vi "MeasureIVandCap.vi"(0 ".NET Refnum in":refnum<k24>, 1 ".NET Refnum":refnum<k24>, 2 "Junction Name":string, 5 "CurrentPositionIndex":i32, 7 "appended path":path, 9 "Numeric":dbl, 12 "new file path (Not A Path if cancelled)":path, 13 "UiDefinition":T1, 14 "Function":string) -> (15 "error out":errorcluster)   [LabVIEW 2020]
uses:
  C:/Users/User/Desktop/Automation/CurrentVersion/LabviewDXFViewer/bin/Release/LabviewDXFViewer.exe
  LabviewDXFViewer/bin/Release/LabviewDXFViewer.exe
  UIReferences.ctl
  <vilib>/Utility/file.llb/Write Delimited Spreadsheet (string).vi
  <vilib>/Utility/file.llb/Write Delimited Spreadsheet (DBL).vi
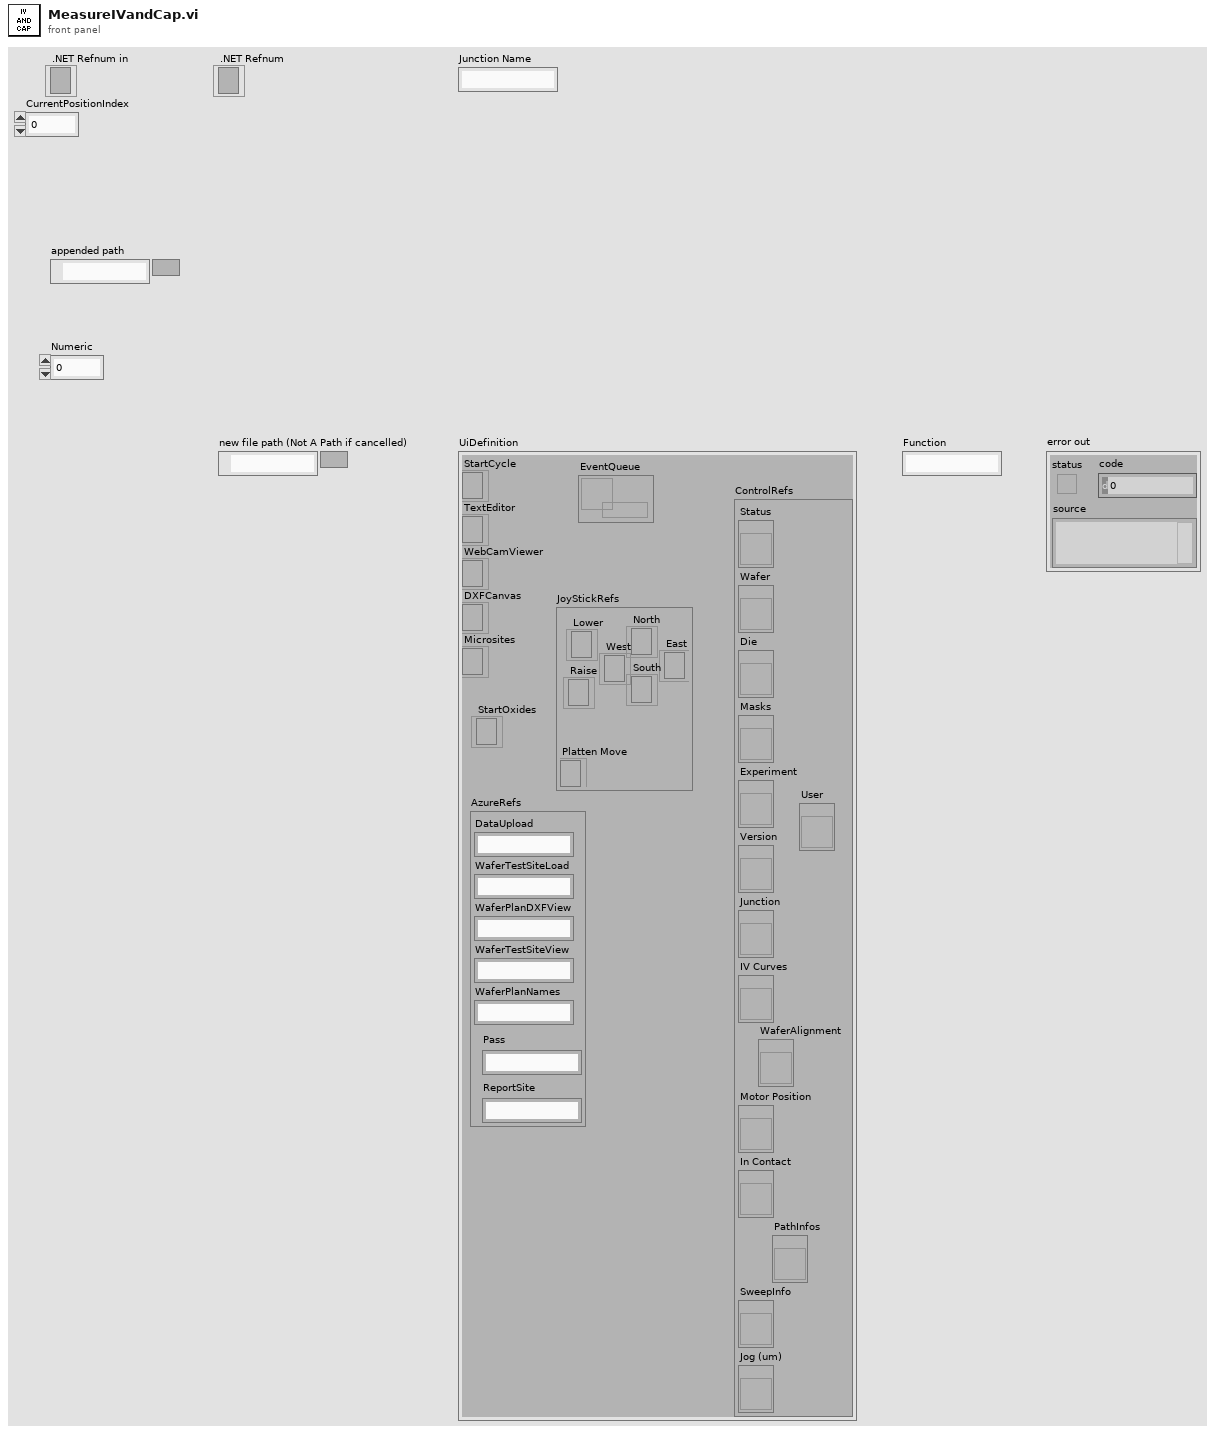
[diagram p1: front panel]
types:
  T1 = typedef "UIReferences.ctl" = cluster{"StartCycle":refnum<k24>, "TextEditor":refnum<k24>, "WebCamViewer":refnum<k24>, "DXFCanvas":refnum<k24>, "Microsites":refnum<k24>, "JoyStickRefs":cluster{"North":refnum<k24>, "Lower":refnum<k24>, "Raise":refnum<k24>, "Platten Move":refnum<k24>, "West":refnum<k24>, "East":refnum<k24>, "South":refnum<k24>}, "AzureRefs":cluster{"DataUpload":string, "WaferTestSiteLoad":string, "WaferPlanDXFView":string, "WaferTestSiteView":string, "WaferPlanNames":string, "Pass":string, "ReportSite":string}, "ControlRefs":cluster{"Status":refnum<vi>, "Wafer":refnum<vi>, "Die":refnum<vi>, "Masks":refnum<vi>, "Experiment":refnum<vi>, "Version":refnum<vi>, "Junction":refnum<vi>, "IV Curves":refnum<vi>, "Motor Position":refnum<vi>, "In Contact":refnum<vi>, "SweepInfo":refnum<vi>, "Jog (um)":refnum<vi>, "PathInfos":refnum<vi>, "User":refnum<vi>, "WaferAlignment":refnum<vi>}, "EventQueue":refnum<queue>, "StartOxides":refnum<k24>}
  T2 = typedef "CapacitanceInfos.ctl" = cluster{"Conductance":dbl, "CapacitanceIV":dbl, "Intercept":dbl, "CapacitanceSW":dbl, "Sum":dbl, "CapacitanceInfos":T3[], "CapacitancePhase":dbl, "dC/dV":dbl, "Function":string, "OtherInfo":dbl[][]}
  T3 = typedef "CapacitanceRecord.ctl" = cluster{"Freq":dbl, "Vpp":dbl, "PhaseS":dbl, "Irms":dbl, "PhaseC":dbl, "Theta":dbl, "VDrive":dbl, "Capacitance":dbl, "Other":dbl}
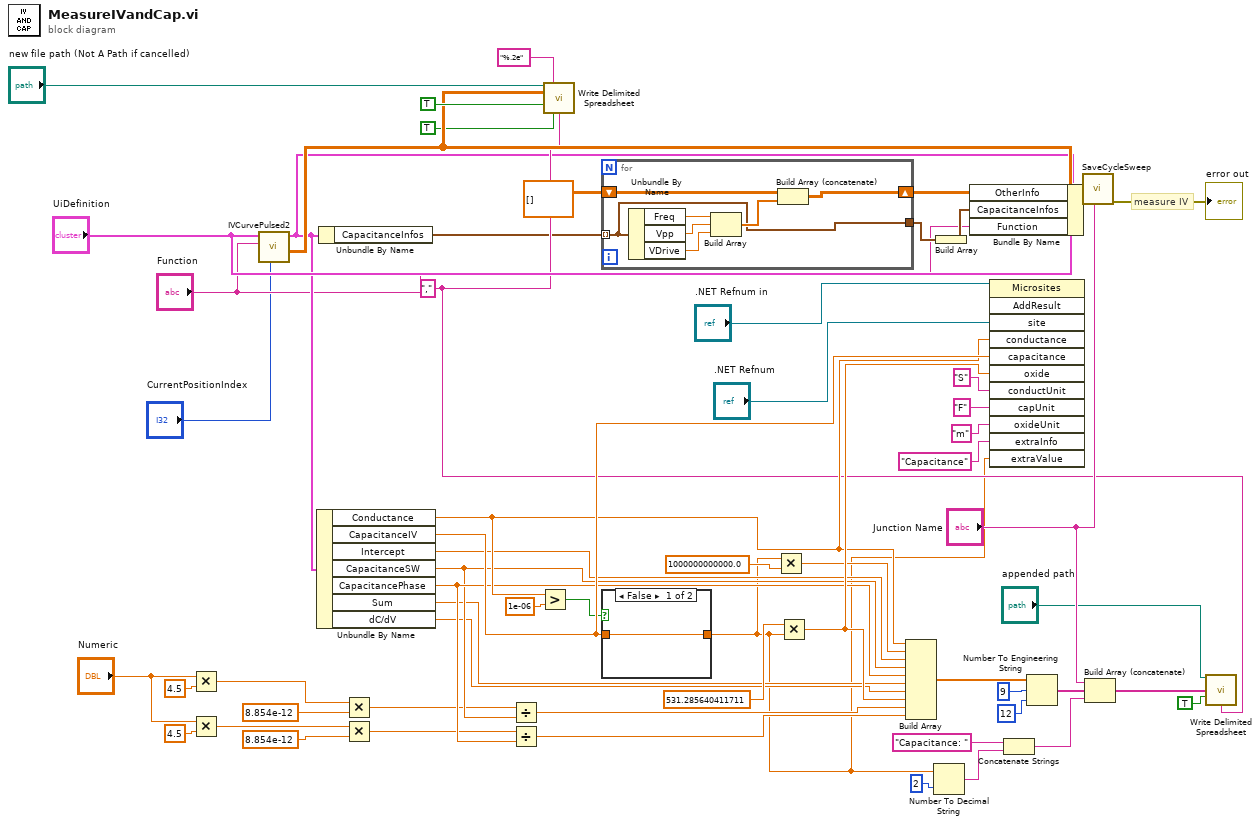
[diagram p0: block diagram]
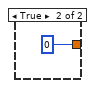
[diagram p2: hidden frame]
diagram:
  w16 = "," ("delimiter (\\t)")
  # "measure IV"
  n1 = Multiply(x="Numeric", y=4.5) -> (x*y=w37:dbl)
  n2 = Multiply(x="Numeric", y=4.5) -> (x*y=w43:dbl)
  n3 = call "IVCurvePulsed2.vi"("CurrentPositionIndex"="CurrentPositionIndex", "Program"="Function", "UiDefinition"="UiDefinition") -> ("appended array"=w27:dbl[][], "InfoCluster"=w9:T2)  [unwired: 7 in]
  n4 = Unbundle By Name(w9) -> ("Conductance"=w57:dbl, "CapacitanceIV"=w58:dbl, "Intercept"=w31:dbl, "CapacitanceSW"=w40:dbl, "CapacitancePhase"=w47:dbl, "Sum"=w32:dbl, "dC/dV"=w33:dbl)
  n5 = Unbundle By Name(w9) -> ("CapacitanceInfos"=w8:T3[])
  n6 = Multiply(x=w37, y=8.854e-12) -> (x*y=w39:dbl)
  n7 = Multiply(x=w43, y=8.854e-12) -> (x*y=w45:dbl)
  n8 = Divide(x=w39, y=w40) -> (x/y=w41:dbl)
  n9 = Divide(x=w45, y=w47) -> (x/y=w48:dbl)
  n10 = Greater?(x=w57, y=1e-06) -> (0:w49:bool)
  n11 = call-poly <vilib>:"Write Delimited Spreadsheet.vi"("file path (dialog if empty)"="new file path (Not A Path if cancelled)", "format (%.3f)"="%.2e", "2D data"=w27, "append to file? (new file:F)"=TRUE, "transpose? (no:F)"=TRUE, "delimiter (\\t)"=w16) -> ()  [unwired: 8 in, 2 out]
  n12 = for {
    tunnel: w8 -> [w61] mode=indexing
    shift-right: [w63] -> w5
    shift-left: dbl[][] [] -> [w62]
    tunnel: [w61] -> w4
    n13 = Unbundle By Name(w61) -> ("Freq"=w67:dbl, "Vpp"=w66:dbl, "VDrive"=w65:dbl)
    n14 = Build Array(w67, w66, w65) -> (w64:dbl[])
    n15 = Build Array (concatenate)(w62, w64) -> (w63:dbl[][])
  }
  n16 = case shown="False" w49 {
    tunnel: [w68 0] -> w12
    tunnel: w58 -> [w68 _]
    frame False {
    }
    frame True {
    }
  }
  n17 = Multiply(x=w12, y=1000000000000.0) -> (x*y=w34:dbl)
  n18 = Multiply(x=531.285640411711, y=w12) -> (x*y=w60:dbl)
  n19 = Build Array(w57, w34, w31, w40, w47, w32, w33, w60, w41, w48) -> (w30:dbl[])
  n20 = Number To Decimal String(number=w12, width (-)=i16 2) -> (decimal integer string=w14:string)
  n21 = Build Array(w4) -> (w3:T3[])
  n22 = Bundle By Name(cluster=w9, "OtherInfo"=w5, "CapacitanceInfos"=w3, "Function"="Function") -> (w6:T2)
  n23 = invoke class="Microsites" method="AddResult"(reference=".NET Refnum in", "site"=".NET Refnum", "conductance"=w57, "capacitance"=w58, "oxide"=w60, "conductUnit"="S", "capUnit"="F", "oxideUnit"="m" ("interceptUnit"), "extraInfo"="Capacitance", "extraValue"=w12) -> ()  [unwired: 2 in, 12 out]
  n24 = Concatenate Strings("Capacitance: ", w14) -> (w10:string)
  n25 = Number To Engineering String(2:i16 12 ("precision (6)"), 3:i16 9 ("width (-)"), 4:w30) -> (0:w21:string[])  [unwired: 1 in]
  n26 = call "SaveCycleSweep.vi"("JunctionName"="Junction Name", "UiDefinition 2"="UiDefinition", "InfoCluster"=w6, "appended array"=w27) -> ("error out"=→"error out":errorcluster)  [unwired: 7 in]
  n27 = Build Array (concatenate)("Junction Name", w21, w10) -> (w23:string[])
  n28 = call-poly <vilib>:"Write Delimited Spreadsheet.vi"("file path (dialog if empty)"="appended path", "1D data"=w23, "append to file? (new file:F)"=TRUE, "delimiter (\\t)"=w16) -> ()  [unwired: 10 in, 2 out]
